vi "Graph.vi"() -> ()   [LabVIEW 2014]
uses:
  <vilib>/Utility/file.llb/Read From Spreadsheet File (DBL).vi
  <vilib>/Utility/file.llb/Read From Spreadsheet File (I64).vi
panel:
  out "Waveform Graph":dbl[][](graph)
  in  "전체_Selected":path
  in  "Selected":path
  in  "W":path
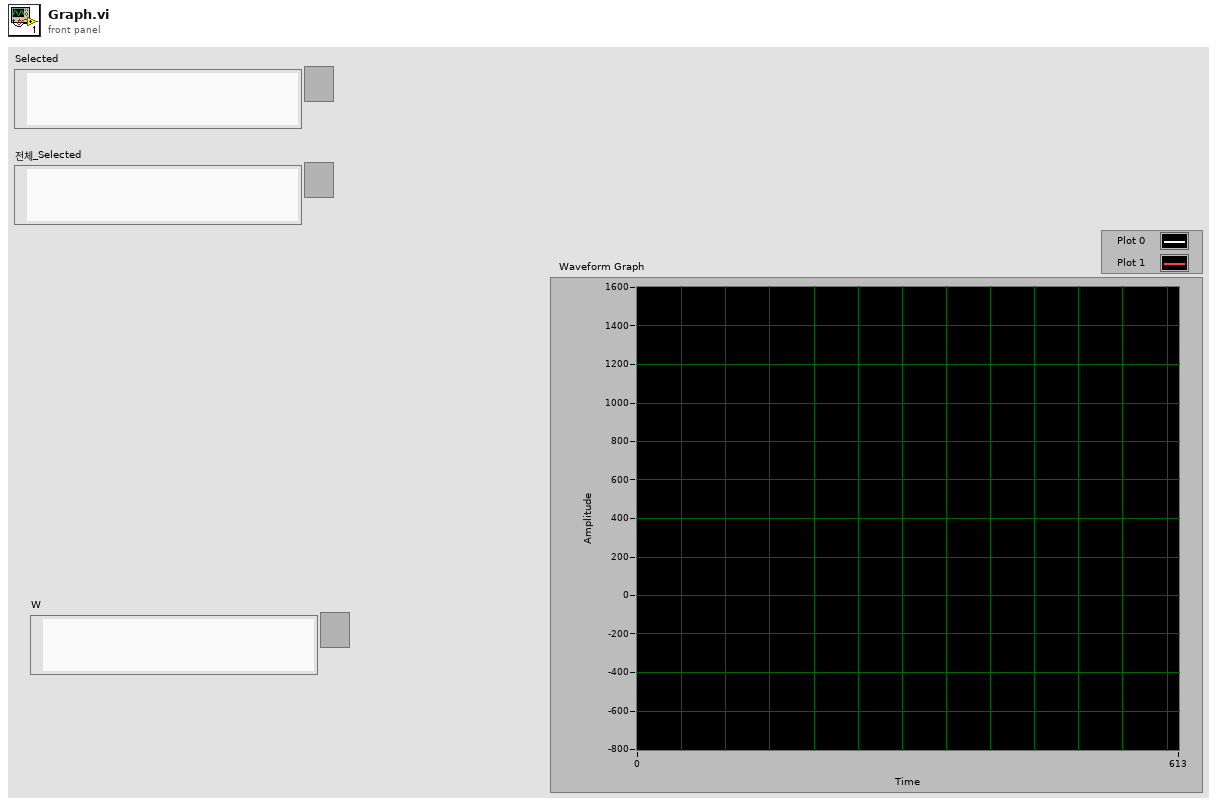
[diagram p1: front panel]
types:
  T1 = enum16{"Transpose", "Vertical Flip", "Horizontal Flip", "Rotate 90", "Rotate 180", "Rotate 270", "Diagonal Flip"}
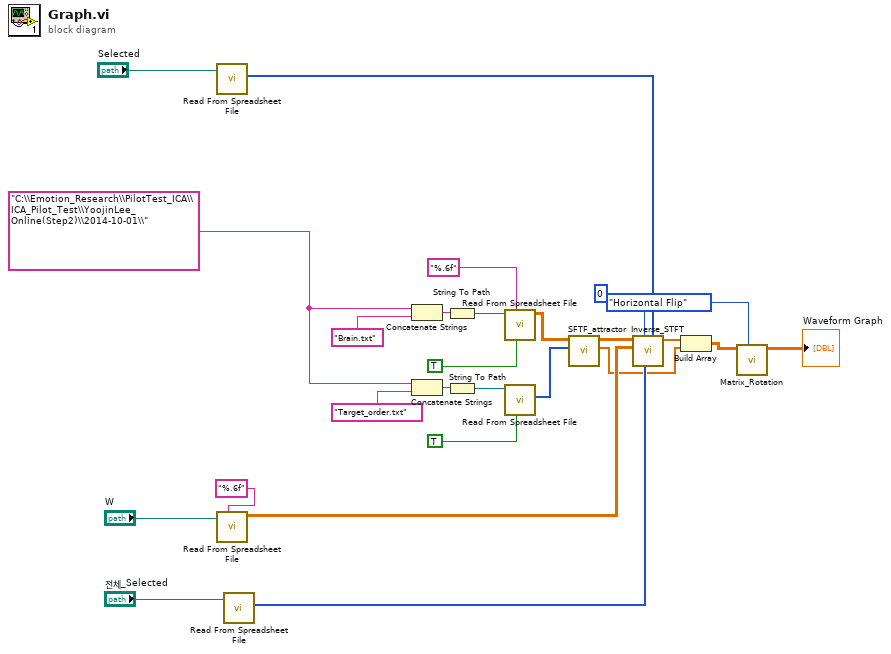
[diagram p0: block diagram]
diagram:
  w6 = "C:\\Emotion_Research\\PilotTest_ICA\\ICA_Pilot_Test\\YoojinLee_Online(Step2)\\2014-10-01\\"
  n1 = call-poly <vilib>:"Read From Spreadsheet File.vi"("file path (dialog if empty)"="Selected") -> ("first row"=w8:i64[])  [unwired: 6 in, 4 out]
  n2 = call-poly <vilib>:"Read From Spreadsheet File.vi"("format (%.3f)"="%.6f", "file path (dialog if empty)"="W") -> ("all rows"=w13:dbl[][])  [unwired: 5 in, 4 out]
  n3 = call-poly <vilib>:"Read From Spreadsheet File.vi"("file path (dialog if empty)"="전체_Selected") -> ("first row"=w9:i64[])  [unwired: 6 in, 4 out]
  n4 = Concatenate Strings(w6, "Brain.txt" ("format (%.3f)")) -> (w23:string)
  n5 = Concatenate Strings(w6, "Target_order.txt" ("format (%.3f)")) -> (w19:string)
  n6 = String To Path(string=w23) -> (path=w22:path)
  n7 = String To Path(string=w19) -> (path=w18:path)
  n8 = call-poly <vilib>:"Read From Spreadsheet File.vi"("transpose (no:F)"=TRUE, "format (%.3f)"="%.6f", "file path (dialog if empty)"=w22) -> ("all rows"=w17:dbl[][])  [unwired: 4 in, 4 out]
  n9 = call-poly <vilib>:"Read From Spreadsheet File.vi"("transpose (no:F)"=TRUE, "file path (dialog if empty)"=w18) -> ("first row"=w16:i64[])  [unwired: 5 in, 4 out]
  n10 = call "SFTF_attractor.vi"("Target_Flash_Order"=w16, "Brain_EEG"=w17) -> ("Non STFT"=w3:dbl[], "STFT Spectrogram {X}"=w15:dbl[][])  [unwired: 8 in]
  n11 = call "Inverse_STFT.vi"("Selected"=w8, "전체_Selected"=w9, "Group Number"=0, "W"=w13, "STFT Spectrogram {X}"=w15) -> ("Inverse_STFT"=w4:dbl[])  [unwired: 6 in]
  n12 = Build Array(w4, w3) -> (w5:dbl[][])
  n13 = call "Matrix_Rotation.vi"("Opt"=T1."Horizontal Flip", "Input"=w5) -> ("Output"=→"Waveform Graph":dbl[][])  [unwired: 9 in]
